vi "CUT_FRT.vi"() -> ()   [LabVIEW 2014]
uses:
  typedefs/eMainAction.ctl
  typedefs/ePathsAction.ctl
  <vilib>/Utility/file.llb/Read From Spreadsheet File (DBL).vi
  <vilib>/Analysis/NI_AALBase.lvlib
panel:
  in  "btnSaveTHD+N":bool
  in  "btnSaveOOBSeq":bool
  in  "Nominal Current":dbl=1.0
  in  "Nominal Voltage":dbl=70.0
  out "OOB Seq":dbl[][](array[numeric]) format="%#.2f"
  in  "btnOOBSeq":bool
  out "THD+N (%)":dbl[][](array[numeric]) format="%#_3f"
  in  "btnFRTAnalysis":bool
  in  "btnExit":bool
  out "error out":errorcluster
  in  "error in (no error)":errorcluster
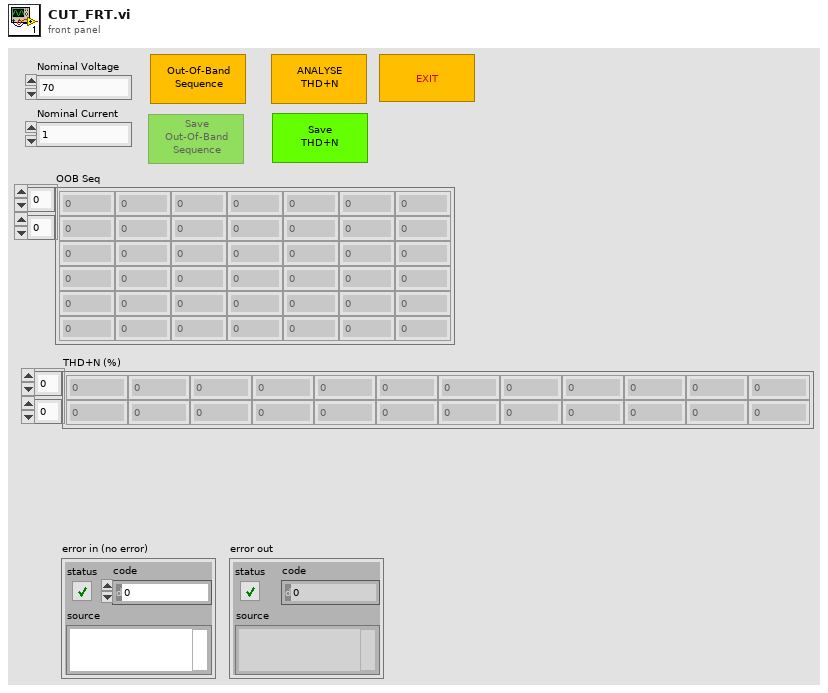
[diagram p1: front panel]
types:
  T1 = enum8{"Enabled", "Disabled", "Disabled and Grayed Out"}
  T2 = typedef "eMainAction.ctl" = enum16{"Init", "ProcessUI", "Exit"}
  T3 = typedef "ePathsAction.ctl" = enum16{"Set", "Get", "Load", "Save", "Default", "Exit"}
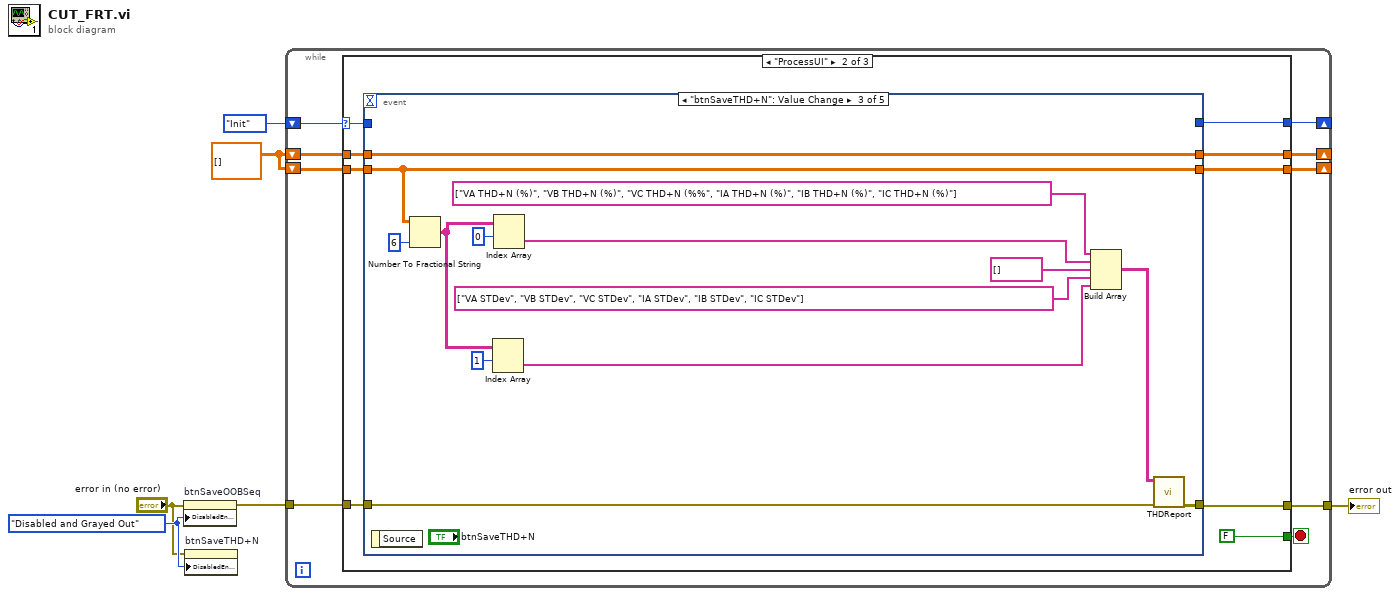
[diagram p0: block diagram]
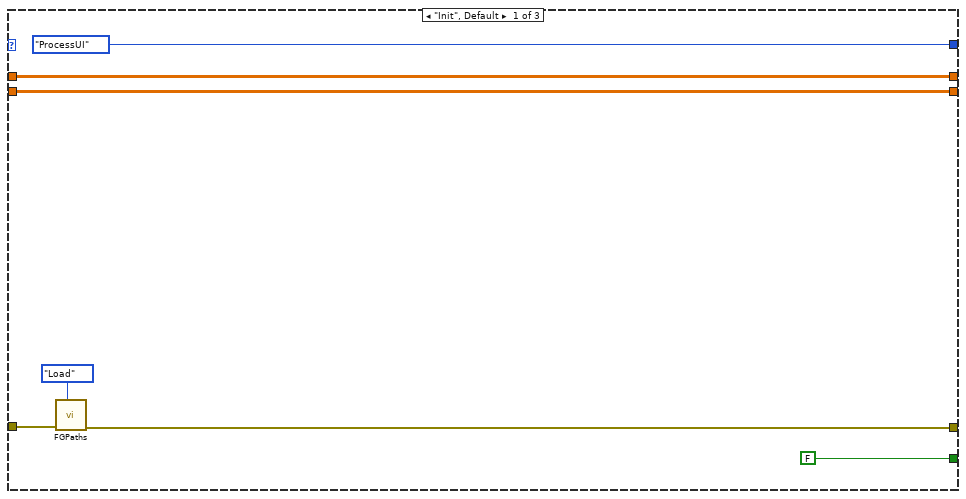
[diagram p2: hidden frame]
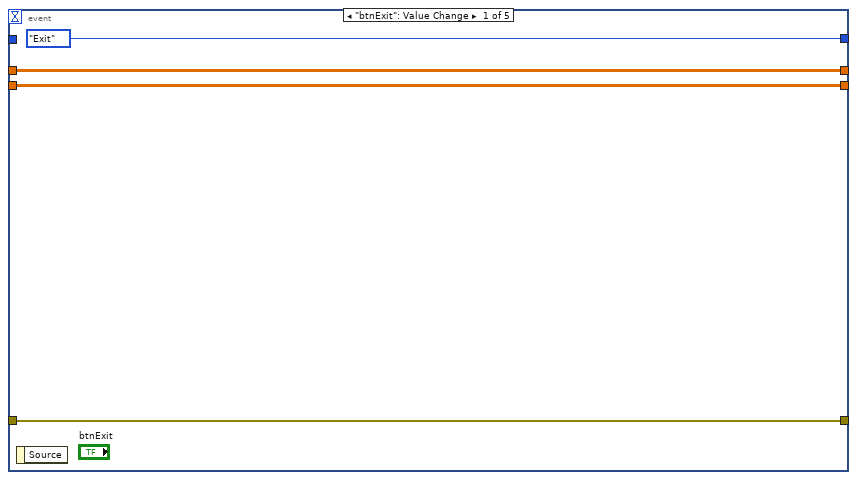
[diagram p3: hidden frame]
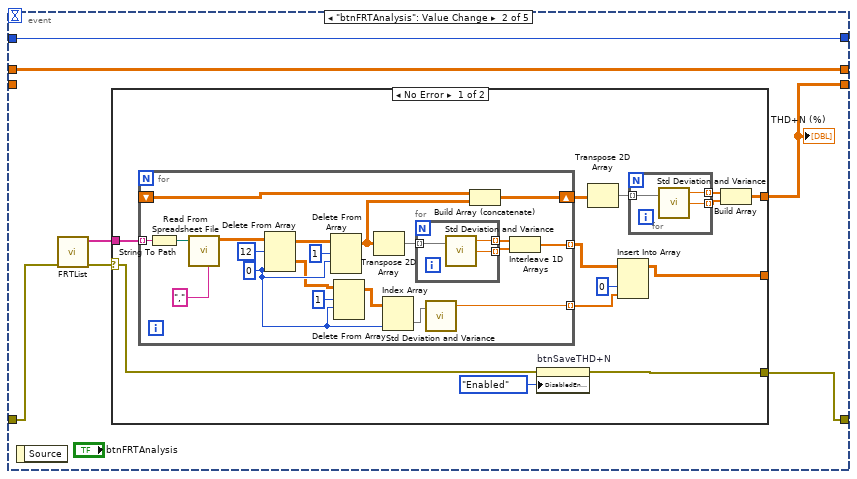
[diagram p4: hidden frame]
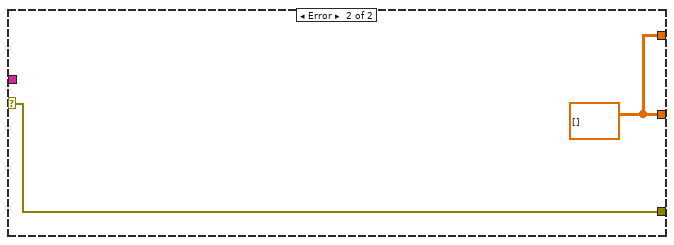
[diagram p5: hidden frame]
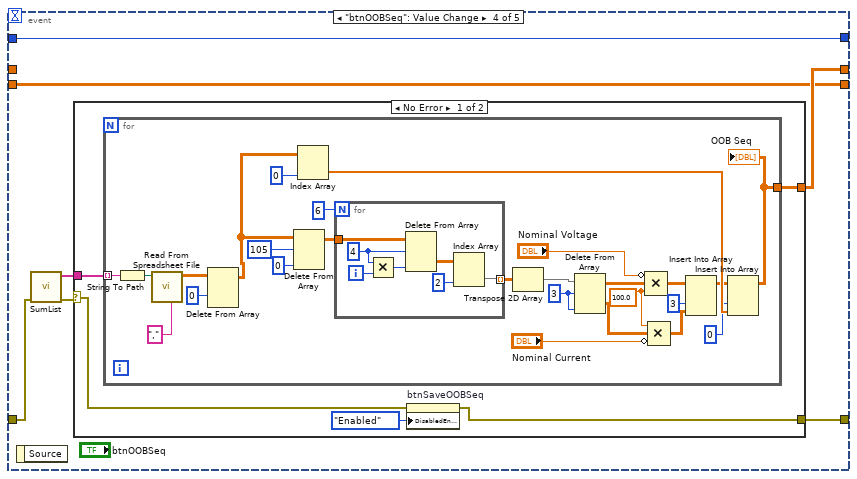
[diagram p6: hidden frame]
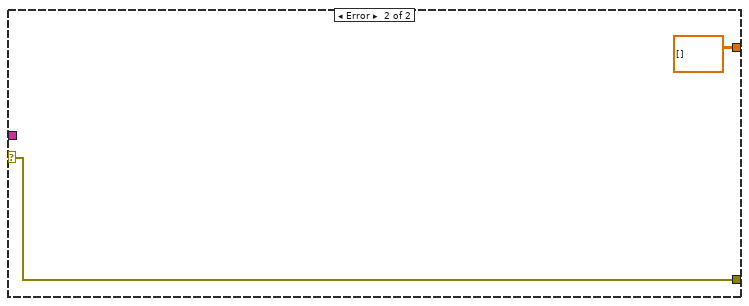
[diagram p7: hidden frame]
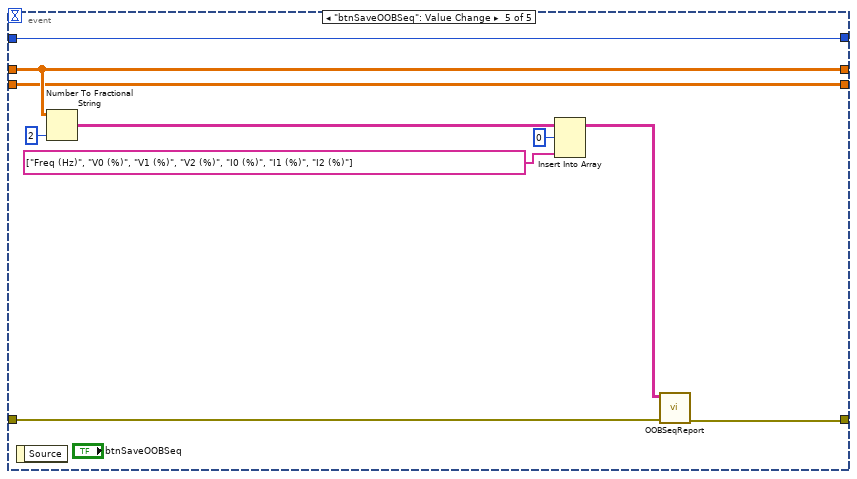
[diagram p8: hidden frame]
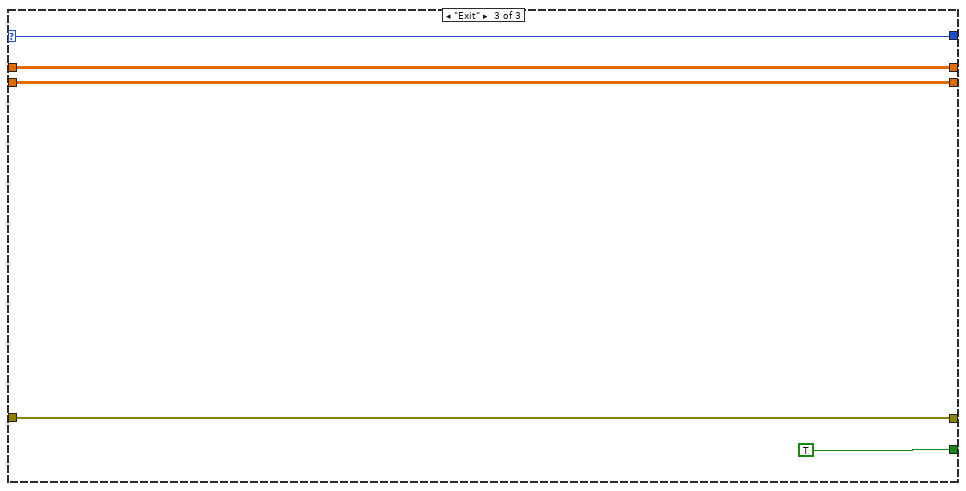
[diagram p9: hidden frame]
diagram:
  w3 = T1."Disabled and Grayed Out" ("Disabled")
  w1 = dbl[][] []
  n1 = property on="btnSaveOOBSeq" class="Bool"(error in="error in (no error)", "DisabledEnum"=w3) -> (error out=w4:errorcluster)  [unwired: 1 in, 1 out]
  n2 = property on="btnSaveTHD+N" class="Bool"(error in="error in (no error)", "DisabledEnum"=w3) -> ()  [unwired: 1 in, 2 out]
  n3 = while {
    tunnel: w4 -> [w13]
    shift-right: [w14] -> _
    shift-left: eMainAction."Init" ("eMainAction") -> [w15]
    tunnel: [w12] -> w5
    shift-right: [w10] -> _
    shift-left: w1 -> [w9]
    shift-right: [w8] -> _
    shift-left: w1 -> [w7]
    stop <- w11 stop-if-true
    n4 = case shown="\"ProcessUI\"" w15 {
      selector: w15 -> [_ w28 w159]
      tunnel: [eMainAction."ProcessUI" ("eMainAction") w31 w159] -> w14
      tunnel: w13 -> [w21 w30 w157]
      tunnel: [w19 w29 w157] -> w12
      tunnel: [FALSE FALSE TRUE] -> w11
      tunnel: [w17 w27 w156] -> w10
      tunnel: w9 -> [w17 w25 w156]
      tunnel: [w16 w24 w155] -> w8
      tunnel: w7 -> [w16 w23 w155]
      frame "Init", Default {
        n5 = call "FGPaths.vi"("ePathsAction"=ePathsAction."Load", "error in (no error)"=w21) -> ("error out"=w19:errorcluster)  [unwired: 8 in, 1 out]
      }
      frame "ProcessUI" {
        n6 = event shown="[2] \"btnSaveTHD+N\": Value Change" {
          selector: _ -> [_ _ _ _ _]
          dyn-events: _ -> [_ _ _ _ _]
          timeout: _ -> [_ _ _ _ _]
          tunnel: [eMainAction."Exit" ("eMainAction") w42 _ w100 w154] -> w31
          tunnel: [w34 w38 w94 w101 w146] -> w29
          tunnel: w30 -> [w34 w41 w93 w104 w148]
          tunnel: w28 -> [_ w42 _ w100 w154]
          tunnel: [w33 w37 w97 w99 w152] -> w27
          tunnel: w25 -> [w33 w37 w97 _ w152]
          tunnel: [w32 w36 w95 w98 w145] -> w24
          tunnel: w23 -> [w32 _ w95 w98 w145]
          event "btnExit": Value Change {
            n7 = event-data() -> ()  [unwired: 1 in, 1 out]
          }
          event "btnFRTAnalysis": Value Change {
            n8 = event-data() -> ()  [unwired: 1 in, 1 out]
            n9 = call "FRTList.vi"("error in (no error)"=w41) -> ("error out"=w39:errorcluster, "FRTList"=w40:string[])  [unwired: 9 in]
            n10 = case shown="No Error" w39 {
              selector: w39 -> [w54 w83]
              tunnel: w40 -> [w55 _]
              tunnel: [w45 w82] -> _
              tunnel: [w53 w83] -> w38
              tunnel: [w43 w82] -> w36
              frame No Error {
                n11 = for {
                  tunnel: w55 -> [w78] mode=indexing
                  tunnel: [w67] -> w44 mode=indexing
                  tunnel: [w66] -> w48 mode=indexing
                  shift-right: [w60] -> w50
                  shift-left: _ -> [w59]
                  w64 = 0 ("disabled index (col)")
                  n12 = String To Path(string=w78) -> (path=w77:path)
                  n13 = call-poly <vilib>:"Read From Spreadsheet File.vi"("delimiter (\\t)"="," ("delimiter (\\t)"), "file path (dialog if empty)"=w77) -> ("all rows"=w75:dbl[][])  [unwired: 5 in, 4 out]
                  n14 = Delete From Array(array=w75, length=12, index (col)=w64) -> (deleted portion=w63:dbl[][], array with subset deleted=w73:dbl[][])  [unwired: 1 in]
                  n15 = Delete From Array(array=w73, length=1, index (row)=w64) -> (array with subset deleted=w61:dbl[][])  [unwired: 1 in, 1 out]
                  n16 = Delete From Array(array=w63, length=1, index (row)=w64) -> (array with subset deleted=w62:dbl[][])  [unwired: 1 in, 1 out]
                  n17 = Transpose 2D Array(2D array=w61) -> (transposed array=w70:dbl[][])
                  n18 = Index Array(array=w62, index (col)=w64) -> (element=w68:dbl[])  [unwired: 1 in]
                  n19 = for {
                    tunnel: w70 -> [w81] mode=indexing
                    tunnel: [w80] -> w71 mode=indexing
                    tunnel: [w79] -> w69 mode=indexing
                    n20 = call <vilib>:"Std Deviation and Variance.vi"("X"=w81) -> ("mean"=w80:dbl, "standard deviation"=w79:dbl)  [unwired: 1 in, 1 out]
                  }
                  n21 = call <vilib>:"Std Deviation and Variance.vi"("X"=w68) -> ("mean"=w66:dbl)  [unwired: 1 in, 2 out]
                  n22 = Build Array (concatenate)(w59, w61) -> (w60:dbl[][])
                  n23 = Interleave 1D Arrays(w71, w69) -> (w67:dbl[])
                }
                n24 = property on="btnSaveTHD+N" class="Bool"(error in=w54, "DisabledEnum"=T1."Enabled" ("Disabled")) -> (error out=w53:errorcluster)  [unwired: 1 in, 1 out]
                n25 = Transpose 2D Array(2D array=w50) -> (transposed array=w49:dbl[][])
                n26 = Insert Into Array(array=w44, index (col)=0 ("disabled index (col)"), new element=w48) -> (w45:dbl[][])  [unwired: 1 in]
                n27 = for {
                  tunnel: w49 -> [w58] mode=indexing
                  tunnel: [w56] -> w47 mode=indexing
                  tunnel: [w57] -> w46 mode=indexing
                  n28 = call <vilib>:"Std Deviation and Variance.vi"("X"=w58) -> ("mean"=w56:dbl, "standard deviation"=w57:dbl)  [unwired: 1 in, 1 out]
                }
                n29 = Build Array(w47, w46) -> (w43:dbl[][])
              }
              frame Error {
                w82 = dbl[][] []
              }
            }
            "THD+N (%)" <- w36
          }
          event "btnSaveTHD+N": Value Change {
            n30 = event-data() -> ()  [unwired: 1 in, 1 out]
            n31 = Number To Fractional String(number=w95, precision (6)=i16 6) -> (F-format string=w92:string[][])  [unwired: 2 in]
            n32 = Index Array(array=w92, index (row)=1) -> (element=w85:string[])  [unwired: 1 in]
            n33 = Index Array(array=w92, index (row)=0) -> (element=w89:string[])  [unwired: 1 in]
            n34 = Build Array(string[] ["VA THD+N (%)", "VB THD+N (%)", "VC THD+N (%%", "IA THD+N (%)", "IB THD+N (%)", "IC THD+N (%)"], w89, string[] [] ("element"), string[] ["VA STDev", "VB STDev", "VC STDev", "IA STDev", "IB STDev", "IC STDev"], w85) -> (w84:string[][])
            n35 = call "THDReport.vi"("error in (no error)"=w93, "THD+N Array"=w84) -> ("error out"=w94:errorcluster)  [unwired: 9 in]
          }
          event "btnOOBSeq": Value Change {
            n36 = event-data() -> ()  [unwired: 1 in, 1 out]
            n37 = call "SumList.vi"("error in (no error)"=w104) -> ("error out"=w103:errorcluster, "SumList"=w102:string[])  [unwired: 9 in]
            n38 = case shown="No Error" w103 {
              selector: w103 -> [w106 w144]
              tunnel: w102 -> [w109 _]
              tunnel: [w107 w144] -> w101
              tunnel: [w108 dbl[][] []] -> w99
              frame No Error {
                n39 = for {
                  tunnel: w109 -> [w135] mode=indexing
                  tunnel: [w110] -> w108
                  w121 = 100.0
                  w126 = 3 ("length")
                  n40 = String To Path(string=w135) -> (path=w134:path)
                  n41 = call-poly <vilib>:"Read From Spreadsheet File.vi"("delimiter (\\t)"="," ("delimiter (\\t)"), "file path (dialog if empty)"=w134) -> ("all rows"=w116:dbl[][])  [unwired: 5 in, 4 out]
                  n42 = Delete From Array(array=w116, index (row)=0) -> (array with subset deleted=w115:dbl[][])  [unwired: 2 in, 1 out]
                  n43 = Delete From Array(array=w115, length=105, index (col)=0 ("disabled index (col)")) -> (array with subset deleted=w129:dbl[][])  [unwired: 1 in, 1 out]
                  n44 = Index Array(array=w115, index (col)=0 ("index (row)")) -> (element=w114:dbl[])  [unwired: 1 in]
                  n45 = for {
                    N: 6 -> [_]
                    tunnel: w129 -> [w142]
                    tunnel: [w136] -> w128 mode=indexing
                    i -> [w141]
                    w139 = 4 ("length")
                    n46 = Multiply(x=w139, y=w141) -> (x*y=w140:i32)
                    n47 = Delete From Array(array=w142, length=w139, index (col)=w140) -> (deleted portion=w138:dbl[][])  [unwired: 1 in, 1 out]
                    n48 = Index Array(array=w138, index (col)=2 ("disabled index (col)")) -> (element=w136:dbl[])  [unwired: 1 in]
                  }
                  n49 = Transpose 2D Array(2D array=w128) -> (transposed array=w117:dbl[][])
                  n50 = Delete From Array(array=w117, length=w126, index (col)=w126) -> (deleted portion=w122:dbl[][], array with subset deleted=w125:dbl[][])  [unwired: 1 in]
                  n51 = Compound Arithmetic op=MULTIPLY(invert "Nominal Voltage", w125, w121) -> (w112:dbl[][])
                  n52 = Compound Arithmetic op=MULTIPLY(w121, w122, invert "Nominal Current") -> (w120:dbl[][])
                  n53 = Insert Into Array(array=w112, index (col)=3 ("disabled index (col)"), new element=w120) -> (w111:dbl[][])  [unwired: 1 in]
                  n54 = Insert Into Array(array=w111, index (col)=0, new element=w114) -> (w110:dbl[][])  [unwired: 1 in]
                  "OOB Seq" <- w110
                }
                n55 = property on="btnSaveOOBSeq" class="Bool"(error in=w106, "DisabledEnum"=T1."Enabled" ("Disabled")) -> (error out=w107:errorcluster)  [unwired: 1 in, 1 out]
              }
              frame Error {
              }
            }
          }
          event "btnSaveOOBSeq": Value Change {
            n56 = event-data() -> ()  [unwired: 1 in, 1 out]
            n57 = Number To Fractional String(number=w152, precision (6)=i16 2) -> (F-format string=w151:string[][])  [unwired: 2 in]
            n58 = Insert Into Array(array=w151, index (row)=0, new element=string[] ["Freq (Hz)", "V0 (%)", "V1 (%)", "V2 (%)", "I0 (%)", "I1 (%)", "I2 (%)"]) -> (w147:string[][])  [unwired: 1 in]
            n59 = call "OOBSeqReport.vi"("error in (no error)"=w148, "Array"=w147) -> ("error out"=w146:errorcluster)  [unwired: 9 in]
          }
        }
      }
      frame "Exit" {
      }
    }
  }
  "error out" <- w5
